vi "Formula Node.vi"() -> ()   [LabVIEW 2020]
panel:
  out "Hipotenusa C":dbl
  in  "CatetoB":dbl
  in  "CatetoA":dbl
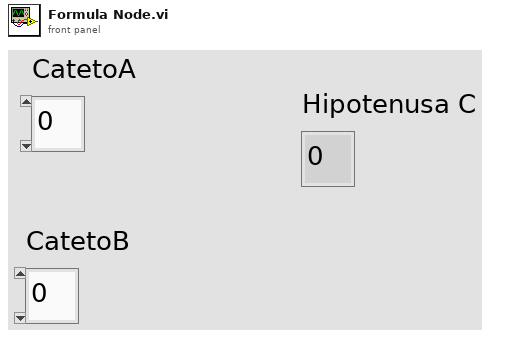
[diagram p1: front panel]
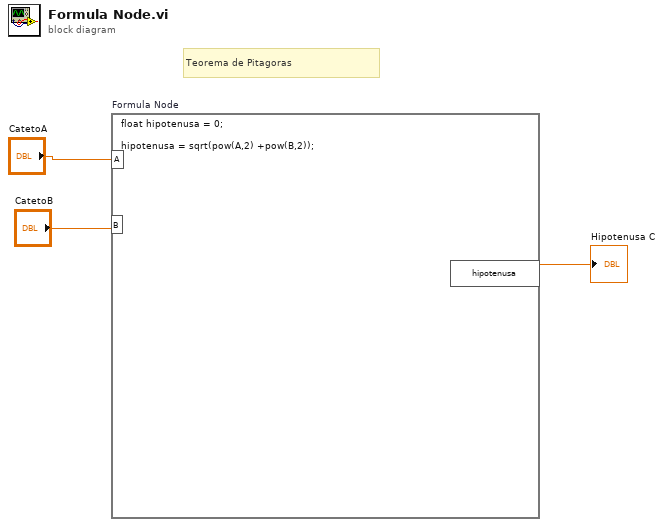
[diagram p0: block diagram]
diagram:
  # "Teorema de Pitagoras"
  n1 = formula code="float hipotenusa = 0;\n\nhipotenusa = sqrt(pow(A,2) +pow(B,2));"("A"="CatetoA", "B"="CatetoB") -> ("hipotenusa"=→"Hipotenusa C":dbl)
